vi "Update Running State.vi"(8 "error in (no error)":errorcluster, 10 "Is Running":bool, 11 "Plugin Session in":refnum<class "Plugin Session.lvclass">) -> (0 "error out":errorcluster, 3 "Plugin Session out":refnum<class "Plugin Session.lvclass">)   [LabVIEW 2023, in "InstrumentStudio Plugin SDK.lvlib" / "Plugin Session.lvclass"]
uses:
  Plugin Session.lvclass
  Plugin Session.lvclass/Plugin Session.ctl
  Read Session Id.vi
  NationalInstruments.VIHost.Interop.dll
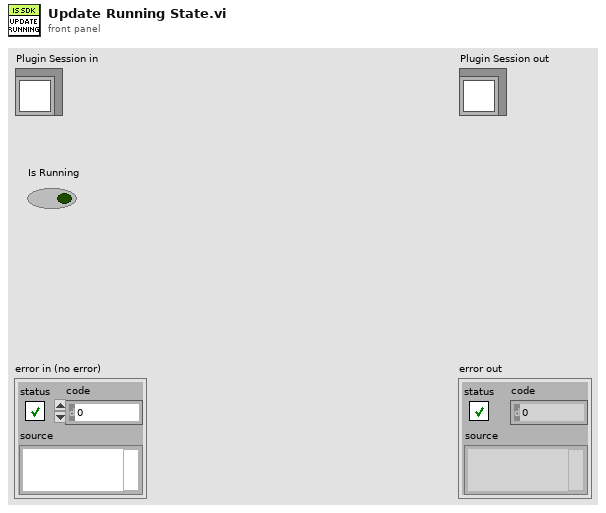
[diagram p1: front panel]
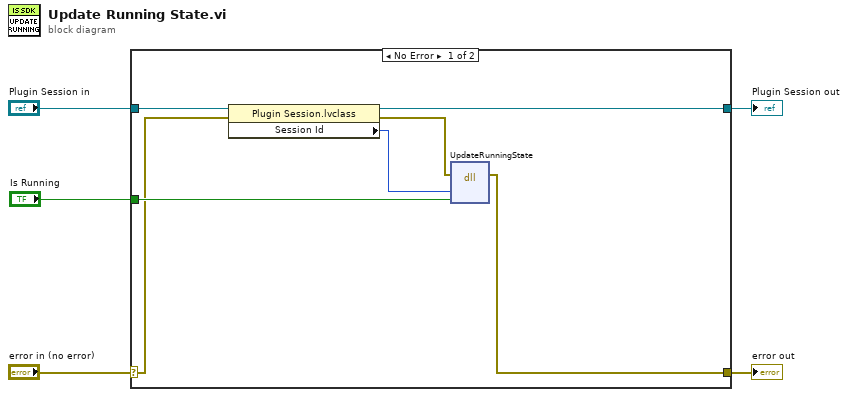
[diagram p0: block diagram]
diagram:
  n1 = case shown="No Error" "error in (no error)" {
    selector: "error in (no error)" -> [w8 w14]
    tunnel: [w6 w14] -> w4
    tunnel: [w10 w13] -> w2
    tunnel: "Plugin Session in" -> [w11 w13]
    tunnel: "Is Running" -> [w12 _]
    frame No Error {
      n2 = property class="Plugin Session.lvclass"(reference=w11, error in=w8) -> (reference out=w10:refnum<class "Plugin Session.lvclass">, error out=w7:errorcluster, "Session Id"=w9:u64)
      n3 = dll-call lib="C:/Users/nmurphy/Downloads/InstrumentStudio_LabVIEW_Plugins/LabVIEW/ExampleProject/PluginSDK/NationalInstruments.VIHost.Interop.dll" fn="UpdateRunningState"(error in=w7, "sessionId"=w9, "isRunning"=w12) -> (error out=w6:errorcluster)  [unwired: 5 in, 1 out]
    }
    frame Error {
    }
  }
  "error out" <- w4
  "Plugin Session out" <- w2
